vi "WEEK.vi"() -> (0 "WEEK":string)   [LabVIEW 2011]
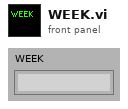
[diagram p1: front panel]
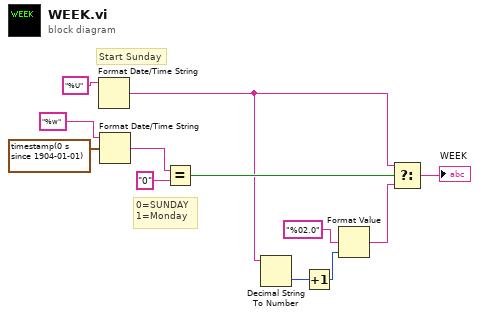
[diagram p0: block diagram]
diagram:
  # "Start Sunday"
  # "0=SUNDAY\n1=Monday"
  n1 = Format Date/Time String(time format string (%c)="%U") -> (date/time string=w2:string)  [unwired: 2 out]
  n2 = Format Date/Time String(time format string (%c)="%w", seconds (now)=timestamp(0 s since 1904-01-01) ("time stamp")) -> (date/time string=w9:string)  [unwired: 1 out]
  n3 = Equal?(x=w9, y="0") -> (x = y?=w5:bool)
  n4 = Decimal String To Number(string=w2) -> (number=w6:i32)  [unwired: 3 out]
  n5 = Increment(x=w6) -> (x+1=w7:i32)
  n6 = Format Value(format string="%02.0", value (0)=w7) -> (output string=w3:string)  [unwired: 1 out]
  n7 = Select(t=w2, s=w5, f=w3) -> (s? t:f=→"WEEK":string)
